vi "Hex to U32.vi"(1 "Hex":string) -> (0 "U32":string)   [LabVIEW 2020, in "Registration.lvclass"]
uses:
  Registration.lvclass
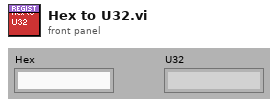
[diagram p1: front panel]
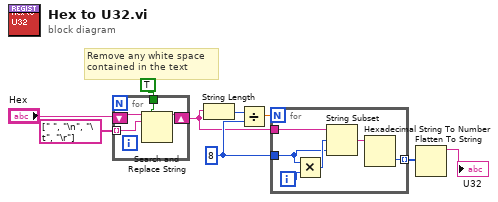
[diagram p0: block diagram]
diagram:
  w7 = 8 ("length (rest)")
  # "Remove any white space\ncontained in the text"
  n1 = for {
    tunnel: TRUE ("replace all? (F)") -> [w13]
    shift-right: [w11] -> w2
    shift-left: "Hex" -> [w12]
    tunnel: string[] [" ", "\n", "\t", "\r"] -> [w10] mode=indexing
    n2 = Search and Replace String(replace all?=w13, input string=w12, search string=w10) -> (result string=w11:string)  [unwired: 5 in, 3 out]
  }
  n3 = String Length(string=w2) -> (length=w5:i32)
  n4 = Divide(x=w5, y=w7) -> (x/y=w6:dbl)
  n5 = for {
    N: w6 -> [_]
    tunnel: w2 -> [w18]
    tunnel: [w19] -> w8 mode=indexing
    tunnel: w7 -> [w14]
    i -> [w16]
    n6 = Multiply(x=w14, y=w16) -> (x*y=w15:i32)
    n7 = String Subset(string=w18, offset (0)=w15, length (rest)=w14) -> (substring=w17:string)
    n8 = Hexadecimal String To Number(string=w17) -> (number=w19:u32)  [unwired: 2 in, 1 out]
  }
  n9 = Flatten To String(anything=w8) -> (data string=→"U32":string)  [unwired: 3 in, 2 out]
